vi "DestroyPrivateEvents.vi"(8 "error in (no error)":errorcluster, 11 "AFM_Litho_Plugin.Data":refnum<class "AFM_Litho_Plugin.Data.lvclass">) -> (0 "error out":errorcluster, 3 "AFM_Litho_Plugin.Data out":refnum<class "AFM_Litho_Plugin.Data.lvclass">)   [LabVIEW 2019, in "AFM_Litho_Plugin.Data.lvclass"]
doc: "JKI State Machine Objects (SMO) 1.0.0.5\nJKI - JKI\nCopyright (c) 2016, JKI"
uses:
  AFM_Litho_Plugin.Data.lvclass
  <vilib>/JKI/JKI SMO/SMO/SMO.lvclass
panel:
  # "For instructions on how to use the JKI State Machine Objects, examples and video tutorials, visit:\nhttp://jki.net/state-machine-objects/\n\nJKI State Machine Objects™\nhttp://jki.net/state-machine-objects/\nCopyright (C) 2005-2015, JKI <info@jki.net>\nALL RIGHTS RESERVED"
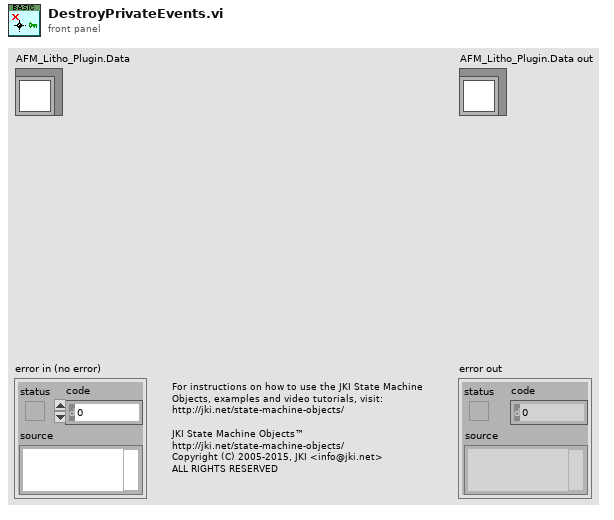
[diagram p1: front panel]
types:
  T1 = typedef "AFM_Litho_Plugin.Data.lvclass/PrivateEvents--Cluster.ctl" = cluster{"SaveSweep":refnum<user-event>}
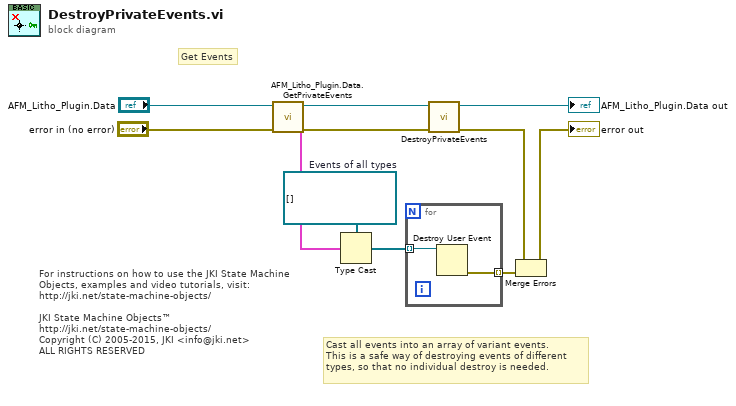
[diagram p0: block diagram]
diagram:
  w7 = refnum<user-event>[] []  # Events of all types
  # "Get Events"
  # "For instructions on how to use the JKI State Machine Objects, examples and video tutorials, visit:\nhttp://jki.net/state-machine-objects/\n\nJKI State Machine Objects™\nhttp://jki.net/state-machine-objects/\nCopyright (C) 2005-2015, JKI <info@jki.net>\nALL RIGHTS RESERVED"
  # "Cast all events into an array of variant events.\nThis is a safe way of destroying events of different\ntypes, so that no individual destroy is needed."
  n1 = call "AFM_Litho_Plugin.Data.GetPrivateEvents.vi"("error in (no error)"="error in (no error)", "AFM_Litho_Plugin.Data"="AFM_Litho_Plugin.Data") -> ("error out"=w4:errorcluster, "Private Events"=w1:T1, "AFM_Litho_Plugin.Data out"=w3:refnum<class "AFM_Litho_Plugin.Data.lvclass">)  [unwired: 7 in]
  n2 = Type Cast(type=w7, x=w1) -> (*(type *) &x=w8:refnum<user-event>[])
  n3 = for {
    tunnel: w8 -> [w13] mode=indexing
    tunnel: [w12] -> w6 mode=indexing
    n4 = Destroy User Event(user event=w13) -> (error out=w12:errorcluster)  [unwired: 1 in]
  }
  n5 = call-parent "DestroyPrivateEvents.vi"("error in (no error)"=w4, "SMO"=w3) -> ("error out"=w10:errorcluster, "SMO out"=→"AFM_Litho_Plugin.Data out":refnum<class "AFM_Litho_Plugin.Data.lvclass">)  [unwired: 8 in]
  n6 = Merge Errors(w10, w6) -> (→"error out":errorcluster)
